vi "Render.vi"(8 "error in (no error)":errorcluster) -> (0 "error out":errorcluster)   [LabVIEW 2021, in "Markdown.lvlib"]
doc: "Render the Library markdown."
uses:
  Markdown.lvlib
  Global.vi
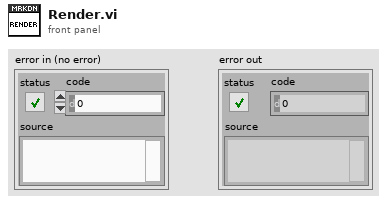
[diagram p1: front panel]
types:
  T1 = typedef "Markdown.lvlib/Item.ctl" = cluster{"Name":string, "Icon":picture, "Path":path, "Title":string, "Desc":string, "ConPane":picture, "TypeString":string, "ProjectItem":string, "VI Type":enum32{"invalid VI type", "Standard VI", "Control VI", "Global VI", "Polymorphic VI", "Configuration VI", "SubSystem", "Facade VI", "Method VI", "Statechart Diagram VI"}}
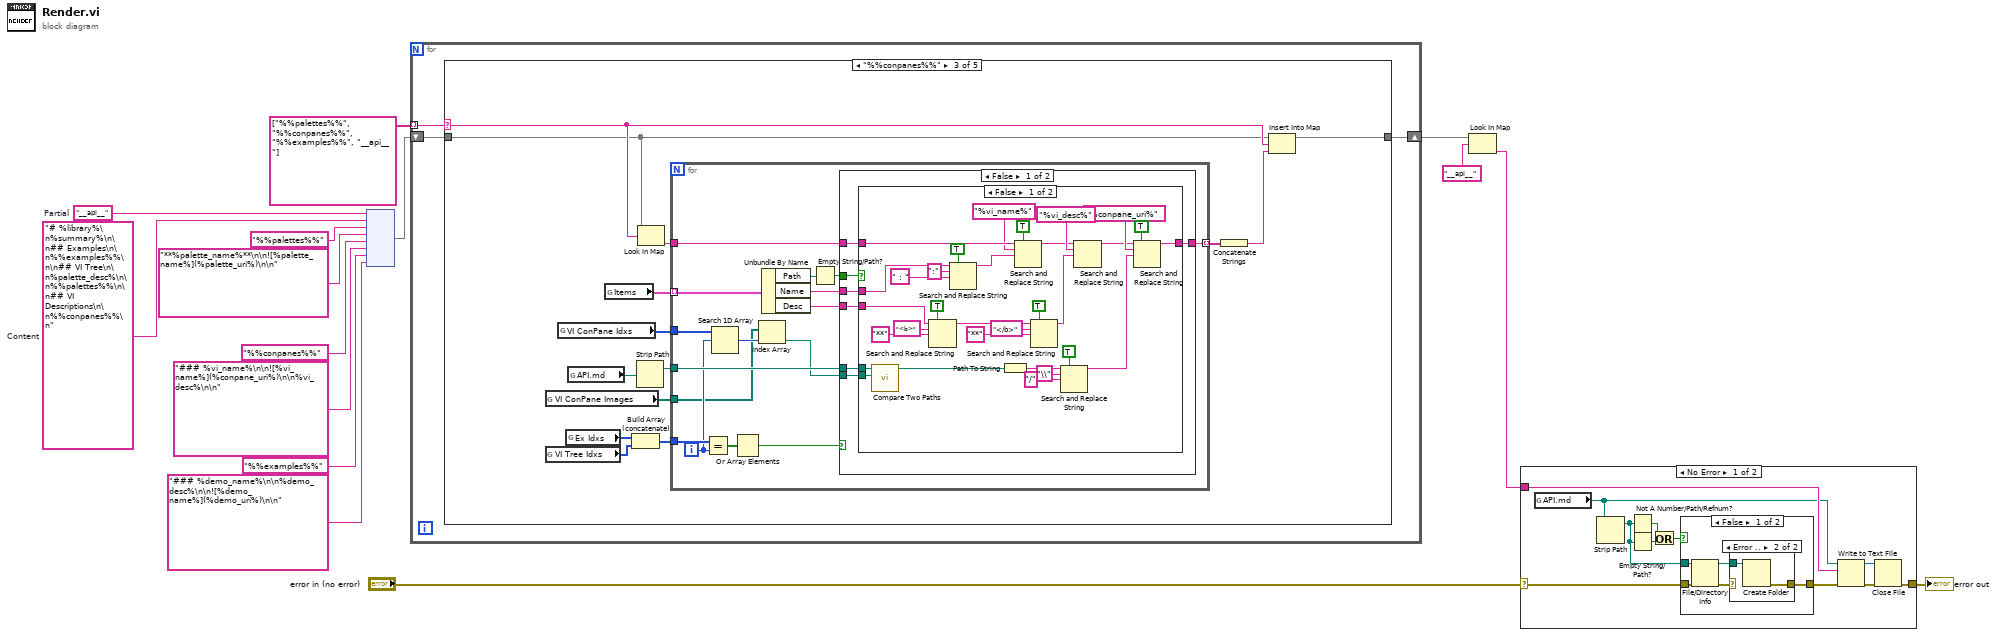
[diagram p0: block diagram]
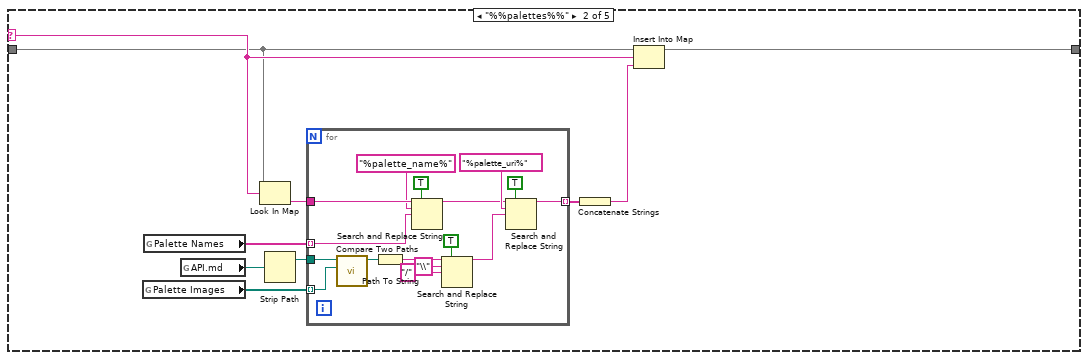
[diagram p6: hidden frame]
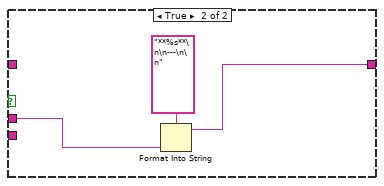
[diagram p7: hidden frame]
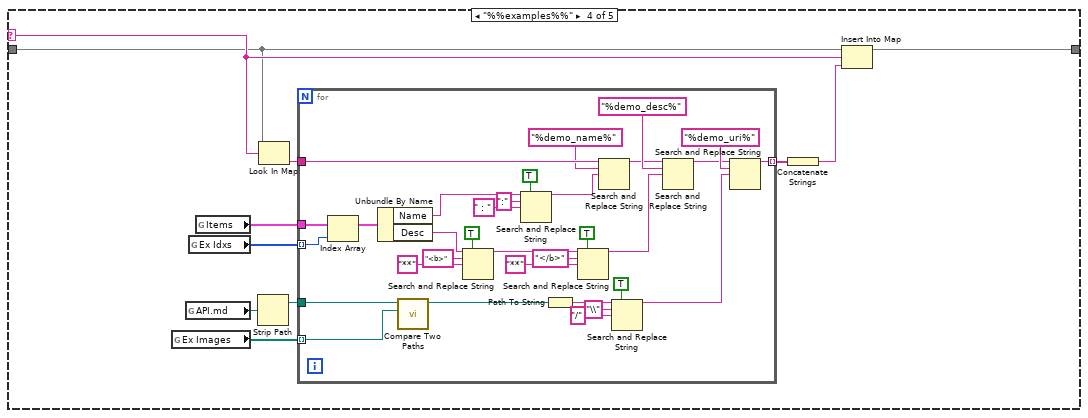
[diagram p9: hidden frame]
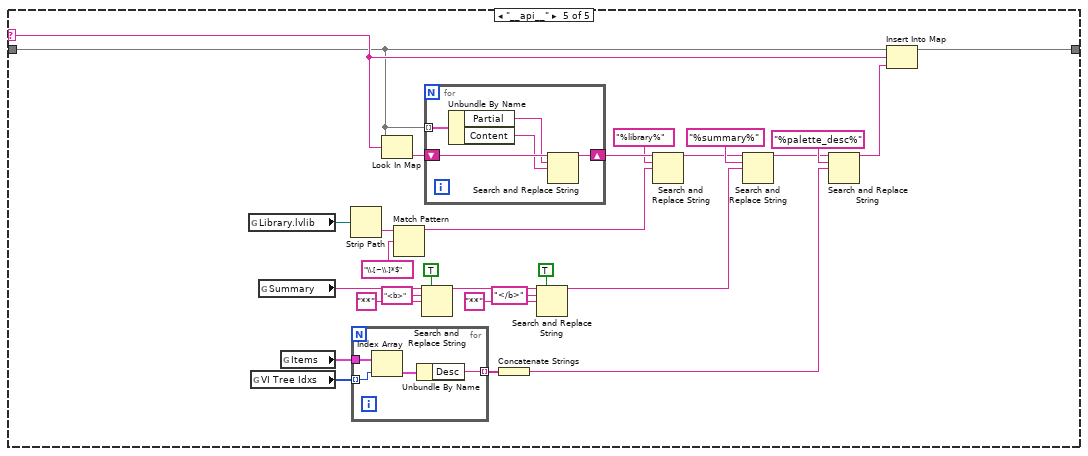
[diagram p10: hidden frame]
diagram:
  w12 = "__api__"  # Partial
  w11 = "# %library%\n%summary%\n\n## Examples\n\n%%examples%%\n\n## VI Tree\n\n%palette_desc%\n\n%%palettes%%\n\n## VI Descriptions\n\n%%conpanes%%\n"  # Content
  n1 = node(w12, w11, "%%palettes%%", "**%palette_name%**\n\n![%palette_name%](%palette_uri%)\n\n", "%%conpanes%%", "### %vi_name%\n\n![%vi_name%](%conpane_uri%)\n\n%vi_desc%\n\n", "%%examples%%", "### %demo_name%\n\n%demo_desc%\n\n![%demo_name%](%demo_uri%)\n\n") -> (w4:map{string, string})
  n2 = for {
    tunnel: string[] ["%%palettes%%", "%%conpanes%%", "%%examples%%", "__api__"] -> [w18] mode=indexing
    shift-right: [w16] -> w2
    shift-left: w4 -> [w17]
    n3 = case shown="\"%%conpanes%%\"" w18 {
      selector: w18 -> [_ w26 w54 w123 w171]
      tunnel: w17 -> [w19 w24 w53 w122 w165]
      tunnel: [w19 w23 w52 w121 w164] -> w16
      frame Default {
      }
      frame "%%palettes%%" {
        n4 = global read "Global.vi" "Palette Images"() -> (w20:path[])
        n5 = global read "Global.vi" "Palette Names"() -> (w22:string[])
        n6 = global read "Global.vi" "API.md"() -> (w21:path)
        n7 = Look In Map(map=w24, key=w26) -> (value=w25:string)  [unwired: 1 in, 1 out]
        n8 = Strip Path(path=w21) -> (stripped path=w27:path)  [unwired: 1 out]
        n9 = for {
          tunnel: w25 -> [w45]
          tunnel: w22 -> [w30] mode=indexing
          tunnel: w27 -> [w43]
          tunnel: w20 -> [w42] mode=indexing
          tunnel: [w38] -> w29 mode=indexing
          n10 = call <vilib>:"Compare Two Paths.vi"("Path 2"=w42, "Path 1"=w43) -> ("Relative Path from 1 to 2"=w39:path)  [unwired: 6 in, 3 out]
          n11 = Path To String(path=w39) -> (string=w36:string)
          n12 = Search and Replace String(replace all?=TRUE ("replace all? (F)"), input string=w45, search string="%palette_name%", replace string=w30) -> (result string=w40:string)  [unwired: 4 in, 3 out]
          n13 = Search and Replace String(replace all?=TRUE ("replace all? (F)"), input string=w36, search string="\\", replace string="/" ("search string")) -> (result string=w33:string)  [unwired: 4 in, 3 out]
          n14 = Search and Replace String(replace all?=TRUE ("replace all? (F)"), input string=w40, search string="%palette_uri%", replace string=w33) -> (result string=w38:string)  [unwired: 4 in, 3 out]
        }
        n15 = Concatenate Strings(w29) -> (w28:string)
        n16 = Insert Into Map(map in=w24, key=w26, value=w28) -> (map out=w23:map{string, string})  [unwired: 2 out]
      }
      frame "%%conpanes%%" {
        n17 = global read "Global.vi" "VI ConPane Images"() -> (w48:path[])
        n18 = global read "Global.vi" "VI Tree Idxs"() -> (w46:i32[])
        n19 = global read "Global.vi" "VI ConPane Idxs"() -> (w50:i32[])
        n20 = global read "Global.vi" "Ex Idxs"() -> (w47:i32[])
        n21 = global read "Global.vi" "API.md"() -> (w49:path)
        n22 = global read "Global.vi" "Items"() -> (w51:T1[])
        n23 = Build Array (concatenate)(w47, w46) -> (w59:i32[])
        n24 = Strip Path(path=w49) -> (stripped path=w58:path)  [unwired: 1 out]
        n25 = Look In Map(map=w53, key=w54) -> (value=w55:string)  [unwired: 1 in, 1 out]
        n26 = for {
          tunnel: w55 -> [w75]
          tunnel: w51 -> [w65] mode=indexing
          tunnel: w58 -> [w73]
          tunnel: w48 -> [w60]
          tunnel: [w72] -> w56 mode=indexing
          tunnel: w59 -> [w68]
          tunnel: w50 -> [w64]
          i -> [w63]
          n27 = Equal?(x=w68, y=w63) -> (x = y?=w67:bool[])
          n28 = Search 1D Array(1D array=w64, element=w63) -> (index of element=w62:i32)  [unwired: 1 in]
          n29 = Or Array Elements(Boolean array=w67) -> (logical OR=w66:bool)
          n30 = Index Array(array=w60, index=w62) -> (element=w61:path)
          n31 = Unbundle By Name(w65) -> ("Path"=w70:path, "Name"=w74:string, "Desc"=w71:string)
          n32 = Empty String/Path?(string/path=w70) -> (empty?=w69:bool)
          n33 = case shown="False" w66 {
            tunnel: w75 -> [w82 _]
            tunnel: w74 -> [w81 _]
            tunnel: w73 -> [w80 _]
            tunnel: w61 -> [w79 _]
            tunnel: [w78 _] -> w72
            tunnel: w71 -> [w77 _]
            tunnel: w69 -> [w76 _]
            frame False {
              n34 = case shown="False" w76 {
                tunnel: w82 -> [w113 _]
                tunnel: w81 -> [w86 w116]
                tunnel: w80 -> [w111 _]
                tunnel: w79 -> [w110 _]
                tunnel: [w108 w115] -> w78
                tunnel: w77 -> [w103 _]
                frame False {
                  n35 = call <vilib>:"Compare Two Paths.vi"("Path 2"=w110, "Path 1"=w111) -> ("Relative Path from 1 to 2"=w91:path)  [unwired: 6 in, 3 out]
                  n36 = Search and Replace String(replace all?=TRUE ("replace all? (F)"), input string=w103, search string="<b>", replace string="**" ("replace string (\"\")")) -> (result string=w97:string)  [unwired: 4 in, 3 out]
                  n37 = Search and Replace String(replace all?=TRUE ("replace all? (F)"), input string=w86, search string=":", replace string=" : " ("replace string (\"\")")) -> (result string=w85:string)  [unwired: 4 in, 3 out]
                  n38 = Path To String(path=w91) -> (string=w94:string)
                  n39 = Search and Replace String(replace all?=TRUE ("replace all? (F)"), input string=w113, search string="%vi_name%", replace string=w85) -> (result string=w106:string)  [unwired: 4 in, 3 out]
                  n40 = Search and Replace String(replace all?=TRUE ("replace all? (F)"), input string=w97, search string="</b>", replace string="**" ("replace string (\"\")")) -> (result string=w96:string)  [unwired: 4 in, 3 out]
                  n41 = Search and Replace String(replace all?=TRUE ("replace all? (F)"), input string=w94, search string="\\", replace string="/" ("search string")) -> (result string=w90:string)  [unwired: 4 in, 3 out]
                  n42 = Search and Replace String(input string=w106, search string="%vi_desc%", replace string=w96) -> (result string=w105:string)  [unwired: 5 in, 3 out]
                  n43 = Search and Replace String(replace all?=TRUE ("replace all? (F)"), input string=w105, search string="%conpane_uri%", replace string=w90) -> (result string=w108:string)  [unwired: 4 in, 3 out]
                }
                frame True {
                  n44 = Format Into String(format string="**%s**\n\n---\n\n" ("result string"), w116) -> (resulting string=w115:string)  [unwired: 2 in, 1 out]
                }
              }
            }
            frame True {
              # "Ignore Example and VI Tree VIs"
            }
          }
        }
        n45 = Concatenate Strings(w56) -> (w57:string)
        n46 = Insert Into Map(map in=w53, key=w54, value=w57) -> (map out=w52:map{string, string})  [unwired: 2 out]
      }
      frame "%%examples%%" {
        n47 = global read "Global.vi" "Ex Images"() -> (w117:path[])
        n48 = global read "Global.vi" "API.md"() -> (w118:path)
        n49 = global read "Global.vi" "Ex Idxs"() -> (w119:i32[])
        n50 = global read "Global.vi" "Items"() -> (w120:T1[])
        n51 = Strip Path(path=w118) -> (stripped path=w124:path)  [unwired: 1 out]
        n52 = Look In Map(map=w122, key=w123) -> (value=w127:string)  [unwired: 1 in, 1 out]
        n53 = for {
          tunnel: w127 -> [w159]
          tunnel: w120 -> [w157]
          tunnel: w124 -> [w156]
          tunnel: w117 -> [w155] mode=indexing
          tunnel: [w153] -> w126 mode=indexing
          tunnel: w119 -> [w133] mode=indexing
          n54 = Index Array(array=w157, index=w133) -> (element=w134:T1)
          n55 = Unbundle By Name(w134) -> ("Name"=w129:string, "Desc"=w148:string)
          n56 = call <vilib>:"Compare Two Paths.vi"("Path 2"=w155, "Path 1"=w156) -> ("Relative Path from 1 to 2"=w136:path)  [unwired: 6 in, 3 out]
          n57 = Search and Replace String(replace all?=TRUE ("replace all? (F)"), input string=w148, search string="<b>", replace string="**" ("replace string (\"\")")) -> (result string=w142:string)  [unwired: 4 in, 3 out]
          n58 = Search and Replace String(replace all?=TRUE ("replace all? (F)"), input string=w129, search string=":", replace string=" : " ("replace string (\"\")")) -> (result string=w128:string)  [unwired: 4 in, 3 out]
          n59 = Path To String(path=w136) -> (string=w139:string)
          n60 = Search and Replace String(replace all?=TRUE ("replace all? (F)"), input string=w142, search string="</b>", replace string="**" ("replace string (\"\")")) -> (result string=w141:string)  [unwired: 4 in, 3 out]
          n61 = Search and Replace String(input string=w159, search string="%demo_name%", replace string=w128) -> (result string=w151:string)  [unwired: 5 in, 3 out]
          n62 = Search and Replace String(replace all?=TRUE ("replace all? (F)"), input string=w139, search string="\\", replace string="/" ("search string")) -> (result string=w135:string)  [unwired: 4 in, 3 out]
          n63 = Search and Replace String(input string=w151, search string="%demo_desc%", replace string=w141) -> (result string=w150:string)  [unwired: 5 in, 3 out]
          n64 = Search and Replace String(input string=w150, search string="%demo_uri%", replace string=w135) -> (result string=w153:string)  [unwired: 5 in, 3 out]
        }
        n65 = Concatenate Strings(w126) -> (w125:string)
        n66 = Insert Into Map(map in=w122, key=w123, value=w125) -> (map out=w121:map{string, string})  [unwired: 2 out]
      }
      frame "__api__" {
        n67 = global read "Global.vi" "Library.lvlib"() -> (w163:path)
        n68 = global read "Global.vi" "VI Tree Idxs"() -> (w160:i32[])
        n69 = global read "Global.vi" "Summary"() -> (w162:string)
        n70 = global read "Global.vi" "Items"() -> (w161:T1[])
        n71 = Strip Path(path=w163) -> (name=w183:string)  [unwired: 1 out]
        n72 = for {
          tunnel: w161 -> [w191]
          tunnel: w160 -> [w190] mode=indexing
          tunnel: [w188] -> w169 mode=indexing
          n73 = Index Array(array=w191, index=w190) -> (element=w189:T1)
          n74 = Unbundle By Name(w189) -> ("Desc"=w188:string)
        }
        n75 = Look In Map(map=w165, key=w171) -> (value=w187:string)  [unwired: 1 in, 1 out]
        n76 = Match Pattern(string=w183, regular expression="\\.[~\\.]*$") -> (before substring=w182:string)  [unwired: 4 out]
        n77 = Search and Replace String(replace all?=TRUE ("replace all? (F)"), input string=w162, search string="<b>", replace string="**" ("replace string (\"\")")) -> (result string=w173:string)  [unwired: 4 in, 3 out]
        n78 = for {
          tunnel: w165 -> [w196] mode=indexing
          shift-right: [w192] -> w186
          shift-left: w187 -> [w195]
          n79 = Unbundle By Name(w196) -> ("Partial"=w194:string, "Content"=w193:string)
          n80 = Search and Replace String(input string=w195, search string=w194, replace string=w193) -> (result string=w192:string)  [unwired: 5 in, 3 out]
        }
        n81 = Concatenate Strings(w169) -> (w168:string)
        n82 = Search and Replace String(replace all?=TRUE ("replace all? (F)"), input string=w173, search string="</b>", replace string="**" ("replace string (\"\")")) -> (result string=w172:string)  [unwired: 4 in, 3 out]
        n83 = Search and Replace String(input string=w186, search string="%library%", replace string=w182) -> (result string=w180:string)  [unwired: 5 in, 3 out]
        n84 = Search and Replace String(input string=w180, search string="%summary%", replace string=w172) -> (result string=w167:string)  [unwired: 5 in, 3 out]
        n85 = Search and Replace String(input string=w167, search string="%palette_desc%", replace string=w168) -> (result string=w166:string)  [unwired: 5 in, 3 out]
        n86 = Insert Into Map(map in=w165, key=w171, value=w166) -> (map out=w164:map{string, string})  [unwired: 2 out]
      }
    }
  }
  n87 = Look In Map(map=w2, key="__api__") -> (value=w1:string)  [unwired: 1 in, 1 out]
  n88 = case shown="No Error" "error in (no error)" {
    selector: "error in (no error)" -> [w200 w217]
    tunnel: [w199 w217] -> w13
    tunnel: w1 -> [w198 _]
    frame No Error {
      n89 = global read "Global.vi" "API.md"() -> (w197:path)
      n90 = Strip Path(path=w197) -> (stripped path=w201:path)  [unwired: 1 out]
      n91 = Not A Number/Path/Refnum?(number/path/refnum=w201) -> (NaN/Path/Refnum?=w204:bool)
      n92 = Empty String/Path?(string/path=w201) -> (empty?=w205:bool)
      n93 = Or(x=w204, y=w205) -> (x .or. y?=w203:bool)
      n94 = case shown="False" w203 {
        tunnel: w200 -> [w212 w216]
        tunnel: [w210 w216] -> w202
        tunnel: w201 -> [w208 _]
        frame False {
          n95 = File/Directory Info(path=w208, error in=w212) -> (path out=w209:path, error out=w211:errorcluster)  [unwired: 5 out]
          n96 = case shown="Error .." w211 {
            selector: w211 -> [w213 _]
            tunnel: [w213 w215] -> w210
            tunnel: w209 -> [_ w214]
            frame No Error {
            }
            frame Error {
              n97 = Create Folder(path (use dialog)=w214) -> (error out=w215:errorcluster)  [unwired: 2 in, 2 out]
            }
          }
        }
        frame True {
        }
      }
      n98 = Write to Text File(file (use dialog)=w197, text=w198, error in=w202) -> (refnum out=w206:refnum<file>, error out=w207:errorcluster)  [unwired: 1 in, 1 out]
      n99 = Close File(refnum=w206, error in=w207) -> (error out=w199:errorcluster)  [unwired: 1 out]
    }
    frame Error {
    }
  }
  "error out" <- w13
